vi "FPGA_controller.vi"() -> ()   [LabVIEW 2017]
uses:
  <vilib>/rvi/Emulation/niFpgaGetClockAttributes.vi
  <vilib>/rvi/Emulation/niFpgaSctlEmulationGetInTimedLoop.vi
  <vilib>/rvi/Emulation/niFpgaEmulationReportErrorSimple.vi
  <vilib>/rvi/eio/common/nirviEmuTemplateMethod_errors.vi
  <vilib>/rvi/Emulation/niFpgaCriticalErrorInLSC.vi
  <vilib>/eio/EIONode/EIONode.xnode
panel:
  out "Translated":i16
  out "VALID":bool
  in  "Scale x2":fxp<+/-,32,16>=10.0 format="%#_21g"
  in  "m_first x2":fxp<+/-,49,33>=4.9499969482421875 format="%#_26g"
  in  "Offset x2":fxp<+/-,48,32> format="%#_26g"
  in  "1/eta x":fxp<+,8,8>=200.0 format="%#_21g"
  in  "m_first x1":fxp<+/-,49,33>=0.649993896484375 format="%#_26g"
  in  "Offset x1":fxp<+/-,48,32> format="%#_26g"
  in  "Scale x1":fxp<+/-,32,16>=5.0 format="%#_21g"
  in  "stop":bool
  # "STATES CONVERSION"
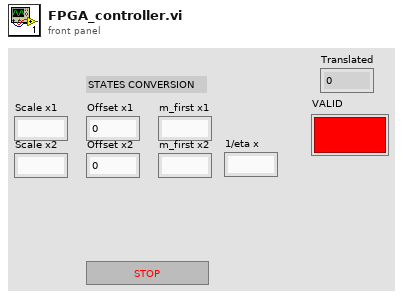
[diagram p1: front panel]
types:
  T1 = cluster{"Boolean array[0]":bool, "Boolean array[1]":bool, "Boolean array[2]":bool, "Boolean array[3]":bool, "Boolean array[4]":bool, "Boolean array[5]":bool, "Boolean array[6]":bool, "Boolean array[7]":bool, "Boolean array[8]":bool, "Boolean array[9]":bool, "Boolean array[10]":bool, "Boolean array[11]":bool, "Boolean array[12]":bool, "Boolean array[13]":bool, "Boolean array[14]":bool, "Boolean array[15]":bool}
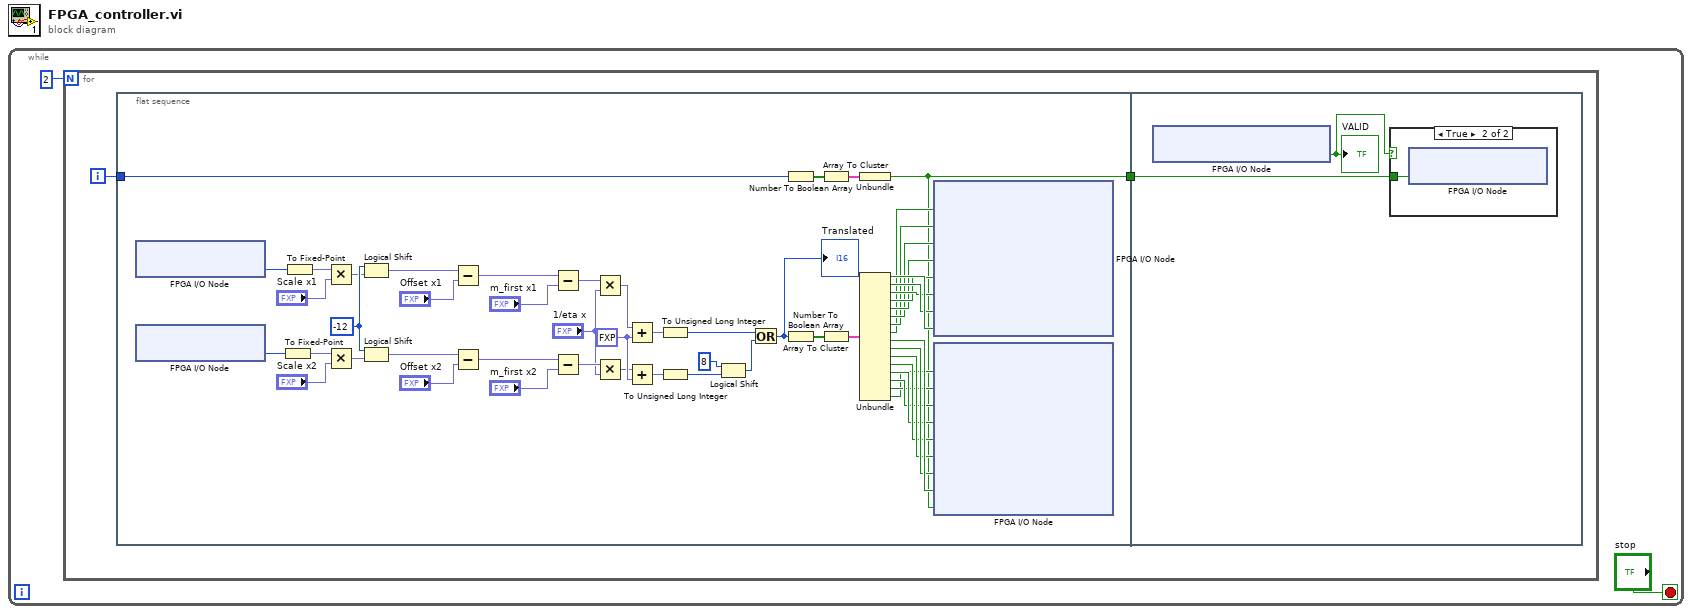
[diagram p0: block diagram]
diagram:
  n1 = while {
    stop <- "stop" stop-if-true
    n2 = for {
      N: 2 -> [_]
      i -> [w4]
      n3 = flat-sequence {
        tunnel: w4 -> [w37]
        tunnel: [w35] -> w3
        tunnel: w3 -> [w58]
        frame #0 {
          w30 = fxp<+,2,1> 0.5 ("y")
          w28 = i16 -12 ("y")
          n4 = xnode "FPGA I/O Node"() -> ("ConnectorA/AI0"=w8:u16)  [unwired: 1 in, 1 out]
          n5 = xnode "FPGA I/O Node"() -> ("ConnectorA/AI1"=w6:u16)  [unwired: 1 in, 1 out]
          n6 = To Fixed-Point(number=w6) -> (fixed-point=w5:fxp<+,16,16>)  [unwired: 1 in]
          n7 = To Fixed-Point(number=w8) -> (fixed-point=w7:fxp<+,16,16>)  [unwired: 1 in]
          n8 = Multiply(x=w7, y="Scale x1") -> (x*y=w27:fxp<+/-,48,32>)
          n9 = Multiply(x=w5, y="Scale x2") -> (x*y=w31:fxp<+/-,48,32>)
          n10 = Logical Shift(y=w28, x=w27) -> (x << y=w24:fxp<+/-,48,32>)
          n11 = Logical Shift(y=w28, x=w31) -> (x << y=w21:fxp<+/-,48,32>)
          n12 = Subtract(x=w24, y="Offset x1") -> (x-y=w25:fxp<+/-,49,33>)
          n13 = Subtract(x=w21, y="Offset x2") -> (x-y=w22:fxp<+/-,49,33>)
          n14 = Subtract(x=w25, y="m_first x1") -> (x-y=w26:fxp<+/-,50,34>)
          n15 = Subtract(x=w22, y="m_first x2") -> (x-y=w20:fxp<+/-,50,34>)
          n16 = Multiply(x=w26, y="1/eta x") -> (x*y=w23:fxp<+/-,58,42>)
          n17 = Multiply(x=w20, y="1/eta x") -> (x*y=w19:fxp<+/-,58,42>)
          n18 = Add(x=w23, y=w30) -> (x+y=w34:fxp<+/-,58,42>)
          n19 = Add(x=w19, y=w30) -> (x+y=w29:fxp<+/-,58,42>)
          n20 = To Unsigned Long Integer(number=w34) -> (unsigned 32bit integer=w11:u32)
          n21 = To Unsigned Long Integer(number=w29) -> (unsigned 32bit integer=w32:u32)
          n22 = Logical Shift(y=8, x=w32) -> (x << y=w10:u32)
          n23 = Or(x=w11, y=w10) -> (x .or. y?=w9:u32)
          "Translated" <- w9
          n24 = Number To Boolean Array(number=w37) -> (Boolean array=w38:bool[])
          n25 = Number To Boolean Array(number=w9) -> (Boolean array=w55:bool[])
          n26 = Array To Cluster(array=w38) -> (cluster=w36:cluster{"Boolean array[0]":bool})
          n27 = Array To Cluster(array=w55) -> (cluster=w56:T1)
          n28 = Unbundle(w36) -> ("Boolean array[0]"=w35:bool)
          n29 = Unbundle(w56) -> ("Boolean array[0]"=w54:bool, "Boolean array[1]"=w53:bool, "Boolean array[2]"=w52:bool, "Boolean array[3]"=w51:bool, "Boolean array[4]"=w50:bool, "Boolean array[5]"=w49:bool, "Boolean array[6]"=w48:bool, "Boolean array[7]"=w47:bool, "Boolean array[8]"=w46:bool, "Boolean array[9]"=w45:bool, "Boolean array[10]"=w44:bool, "Boolean array[11]"=w43:bool, "Boolean array[12]"=w42:bool, "Boolean array[13]"=w41:bool, "Boolean array[14]"=w40:bool, "Boolean array[15]"=w39:bool)
          n30 = xnode "FPGA I/O Node"("Component-Level IP\\pi00"=w47, "Component-Level IP\\pi01"=w48, "Component-Level IP\\pi02"=w49, "Component-Level IP\\pi03"=w50, "Component-Level IP\\pi04"=w51, "Component-Level IP\\pi05"=w52, "Component-Level IP\\pi06"=w53, "Component-Level IP\\pi07"=w54) -> ()  [unwired: 8 in, 8 out]
          n31 = xnode "FPGA I/O Node"("Component-Level IP\\pi08"=w39, "Component-Level IP\\pi09"=w40, "Component-Level IP\\pi10"=w41, "Component-Level IP\\pi11"=w42, "Component-Level IP\\pi12"=w43, "Component-Level IP\\pi13"=w44, "Component-Level IP\\pi14"=w45, "Component-Level IP\\pi15"=w46, "Component-Level IP\\pi16"=w35) -> ()  [unwired: 9 in, 9 out]
        }
        frame #1 {
          n32 = xnode "FPGA I/O Node"() -> ("Component-Level IP\\po0"=w57:bool)  [unwired: 1 in, 1 out]
          "VALID" <- w57
          n33 = case shown="True" w57 {
            tunnel: w58 -> [_ w59]
            frame False {
            }
            frame True {
              n34 = xnode "FPGA I/O Node"("ConnectorA/DIO0"=w59) -> ()  [unwired: 1 in, 1 out]
            }
          }
        }
      }
    }
  }
